vi "Bubble Sort.vi"(8 "Sorting":T1(ring), 11 "list in in":T2[](array[typedef]) {"Creation Date" format="%<%x>T"; "Last Updated" format="%<%x>T"}) -> (3 "list out":T2[](array[typedef]) {"Creation Date" format="%<%x>T"; "Last Updated" format="%<%x>T"})   [LabVIEW 2018]
uses:
  Type Defs/SR Cluster.ctl
  Type Defs/SR Status.ctl
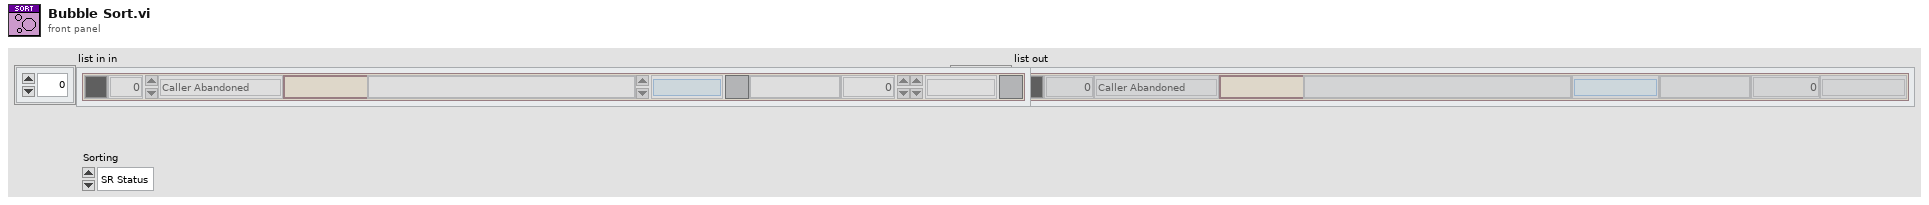
[diagram p1: front panel]
types:
  T1 = enum16{"SR Status", "Most Recent", "SR Type", "SR Number"}
  T2 = typedef "SR Cluster.ctl" = cluster{"Color":u32, "SR Number":i32, "SR Status":T3, "SR Type":string, "Summary":string, "Last Updated":timestamp, "Service Level":string, "Days Open":dbl, "Creation Date":timestamp}
  T3 = typedef "SR Status.ctl" = enum16{"Caller Abandoned", "Created in Error", "Expired", "Forum Resolved AE", "Forum Resolved Customer", "IN WORK", "IN WORK Collab with AES", "IN WORK Collab with PSE", "IN WORK Collab with SE", "IN WORK Customer Added Note", "IN WORK Escalation", "IN WORK Wait on Customer", "Open", "Potentially Resolved", "Presumed Resolved", "RMA Approved for Return", "Resolved", "Passed Off"}
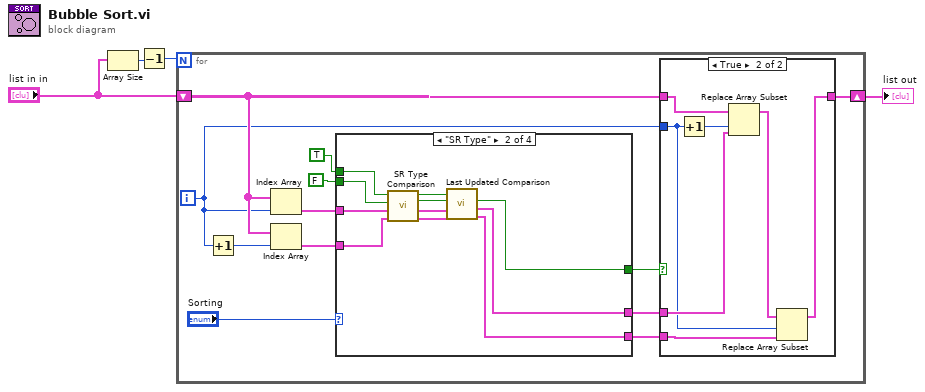
[diagram p0: block diagram]
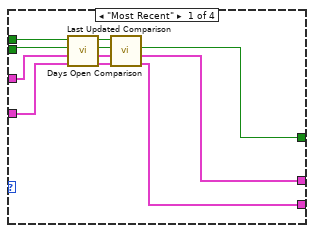
[diagram p2: hidden frame]
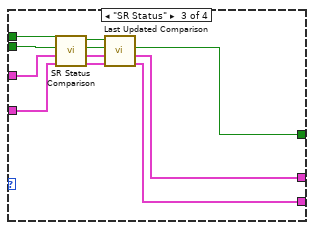
[diagram p3: hidden frame]
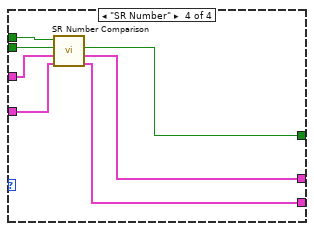
[diagram p4: hidden frame]
diagram:
  n1 = Array Size(array="list in in") -> (size(s)=w2:i32)
  n2 = Decrement(x=w2) -> (x-1=w1:i32)
  n3 = for {
    N: w1 -> [_]
    shift-right: [w11] -> w4
    shift-left: "list in in" -> [w12]
    i -> [w7]
    n4 = Increment(x=w7) -> (x+1=w16:i32)
    n5 = Index Array(array=w12, index=w7) -> (element=w13:T2)
    n6 = Index Array(array=w12, index=w16) -> (element=w14:T2)
    n7 = case shown="\"SR Type\"" "Sorting" {
      tunnel: w14 -> [w24 w35 w46 w53]
      tunnel: w13 -> [w25 w36 w47 w54]
      tunnel: [w18 w28 w40 w51] -> w10
      tunnel: [w17 w29 w41 w50] -> w9
      tunnel: [w19 w30 w39 w52] -> w8
      tunnel: TRUE ("equal? in") -> [w27 w38 w48 w56]
      tunnel: FALSE ("flip? in") -> [w26 w37 w49 w55]
      frame "Most Recent" {
        n8 = call "Last Updated Comparison.vi"("SR Cluster 2 in"=w24, "SR Cluster 1 in"=w25, "flip? in"=w26, "equal? in"=w27) -> ("SR Cluster 2 out"=w20:T2, "SR Cluster 1 out"=w21:T2, "flip? out"=w22:bool, "equal? out"=w23:bool)  [unwired: 4 in]
        n9 = call "Days Open Comparison.vi"("SR Cluster 2 in"=w20, "SR Cluster 1 in"=w21, "flip? in"=w22, "equal? in"=w23) -> ("SR Cluster 2 out"=w17:T2, "SR Cluster 1 out"=w18:T2, "flip? out"=w19:bool)  [unwired: 4 in, 1 out]
      }
      frame "SR Type" {
        n10 = call "SR Type Comparison.vi"("SR Cluster 2 in"=w35, "SR Cluster 1 in"=w36, "flip? in"=w37, "equal? in"=w38) -> ("SR Cluster 2 out"=w34:T2, "SR Cluster 1 out"=w33:T2, "flip? out"=w32:bool, "equal? out"=w31:bool)  [unwired: 4 in]
        n11 = call "Last Updated Comparison.vi"("SR Cluster 2 in"=w34, "SR Cluster 1 in"=w33, "flip? in"=w32, "equal? in"=w31) -> ("SR Cluster 2 out"=w29:T2, "SR Cluster 1 out"=w28:T2, "flip? out"=w30:bool)  [unwired: 4 in, 1 out]
      }
      frame "SR Status" {
        n12 = call "SR Status Comparison.vi"("SR Cluster 2 in"=w46, "SR Cluster 1 in"=w47, "flip? in"=w49, "equal? in"=w48) -> ("SR Cluster 2 out"=w42:T2, "SR Cluster 1 out"=w43:T2, "flip? out"=w44:bool, "equal? out"=w45:bool)  [unwired: 4 in]
        n13 = call "Last Updated Comparison.vi"("SR Cluster 2 in"=w42, "SR Cluster 1 in"=w43, "flip? in"=w44, "equal? in"=w45) -> ("SR Cluster 2 out"=w41:T2, "SR Cluster 1 out"=w40:T2, "flip? out"=w39:bool)  [unwired: 4 in, 1 out]
      }
      frame "SR Number" {
        n14 = call "SR Number Comparison.vi"("SR Cluster 2 in"=w53, "SR Cluster 1 in"=w54, "flip? in"=w55, "equal? in"=w56) -> ("SR Cluster 2 out"=w50:T2, "SR Cluster 1 out"=w51:T2, "flip? out"=w52:bool)  [unwired: 4 in, 1 out]
      }
    }
    n15 = case shown="True" w8 {
      tunnel: w12 -> [w57 w63]
      tunnel: [w57 w58] -> w11
      tunnel: w10 -> [_ w60]
      tunnel: w9 -> [_ w62]
      tunnel: w7 -> [_ w59]
      frame False {
      }
      frame True {
        n16 = Increment(x=w59) -> (x+1=w64:i32)
        n17 = Replace Array Subset(array=w63, new element=w60, index=w64) -> (w61:T2[])
        n18 = Replace Array Subset(array=w61, new element=w62, index=w59) -> (w58:T2[])
      }
    }
  }
  "list out" <- w4
